vi "例5.15 生成一段正弦波形并获得它的波形成分.vi"() -> ()   [LabVIEW 2017]
uses:
  <vilib>/measure/NI_MABase.lvlib
panel:
  out "波形图":waveform(dbl)(graph)
  in  "采样信息":cluster{"Fs":dbl, "#s":dbl}={"Fs"=1000.0, "#s"=1000.0} {"Fs" format="%.2p"}
  in  "相位":dbl format="%.2p"
  in  "幅值":dbl=1.0 format="%0.2p"
  in  "频率":dbl=10.0 format="%0.2p"
  out "dt":dbl
  out "Y":dbl[](array[numeric])
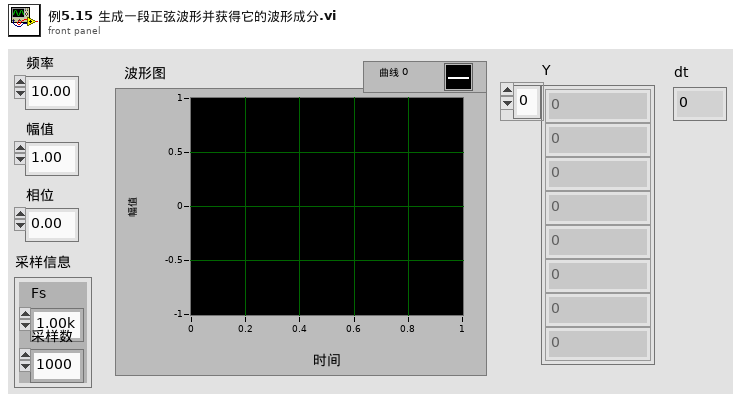
[diagram p1: front panel]
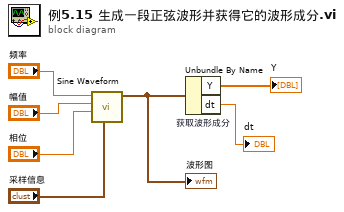
[diagram p0: block diagram]
diagram:
  n1 = call <vilib>:"Sine Waveform.vi"("sampling info"="采样信息", "phase"="相位", "amplitude"="幅值", "frequency"="频率") -> ("signal out"=w1:waveform(dbl))  [unwired: 6 in, 1 out]
  "波形图" <- w1
  n2 = Unbundle By Name "获取波形成分"(w1) -> ("Y"=→"Y":dbl[], "dt"=→"dt":dbl)
